vi "Get SMO RC Type.vi"(8 "error in (no error)":errorcluster, 11 "Inst.Krohn-Hite-7008Instrument in":refnum<class "Inst.Krohn-Hite-7008.lvclass">) -> (0 "error out":errorcluster, 2 "RemoteControl":refnum<class "RemoteControl.lvclass">, 3 "Inst.Krohn-Hite-7008Instrument out":refnum<class "Inst.Krohn-Hite-7008.lvclass">)   [LabVIEW 2019, in "Inst.Krohn-Hite-7008.lvclass"]
uses:
  Inst.Krohn-Hite-7008.lvclass
  <userlib>/LevyLab/Instrument Framework/Instrument Types/VSource/Instrument.VSource.lvclass
  <userlib>/LevyLab/RemoteControl/RemoteControl.lvclass
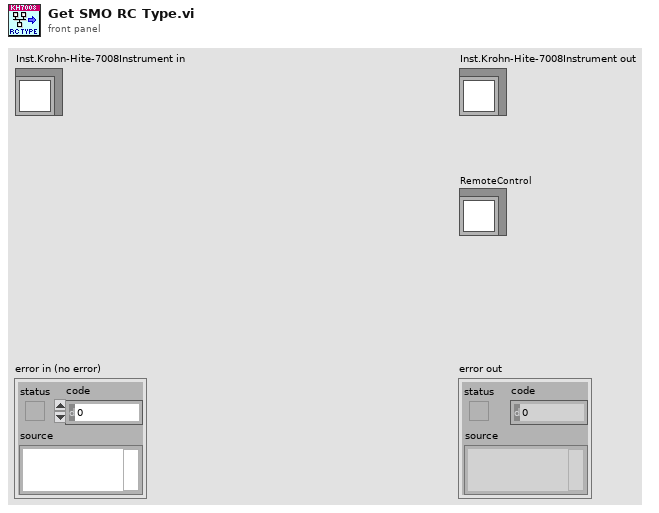
[diagram p1: front panel]
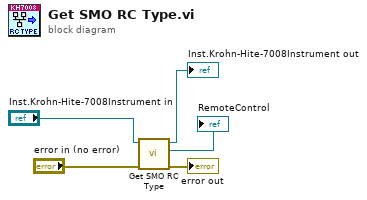
[diagram p0: block diagram]
diagram:
  n1 = call-parent "Get SMO RC Type.vi"("error in (no error)"="error in (no error)", "Instrument in"="Inst.Krohn-Hite-7008Instrument in") -> ("error out"=→"error out":errorcluster, "RemoteControl"=→"RemoteControl":refnum<class "RemoteControl.lvclass">, "Instrument out"=→"Inst.Krohn-Hite-7008Instrument out":refnum<class "Inst.Krohn-Hite-7008.lvclass">)  [unwired: 7 in]
